vi "1_2.vi"() -> ()   [LabVIEW 2010]
panel:
  in  "OK Button":bool
  out "Numeric":i32
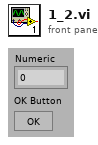
[diagram p1: front panel]
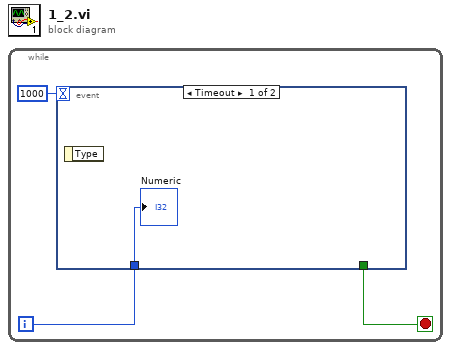
[diagram p0: block diagram]
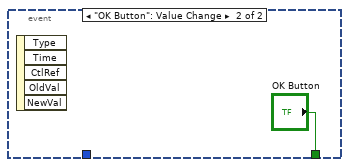
[diagram p2: hidden frame]
diagram:
  n1 = while {
    i -> [w1]
    stop <- w2 stop-if-true
    n2 = event shown="[0] Timeout" {
      selector: _ -> [_ _]
      dyn-events: _ -> [_ _]
      timeout: 1000 -> [_ _]
      tunnel: [_ "OK Button"] -> w2
      tunnel: w1 -> [w4 _]
      event Timeout {
        n3 = event-data() -> ()  [unwired: 1 in, 1 out]
        "Numeric" <- w4
      }
      event "OK Button": Value Change {
        n4 = event-data() -> ()  [unwired: 1 in, 5 out]
      }
    }
  }
